vi "DIO.vi"() -> ()   [LabVIEW 2019]
uses:
  <userlib>/DAQNavi Polymorphic VI/create/DAQNavi Create Channel(DO-Digital Output).vi
  <userlib>/DAQNavi Polymorphic VI/create/DAQNavi Create Channel(DI-Digital Input).vi
  <userlib>/DAQNavi Polymorphic VI/create/DAQNavi Create Channel(AI-Voltage).vi
  <vilib>/measure/mamon.llb/Trigger Detection for 1 Channel.vi
  <userlib>/DAQNavi Polymorphic VI/read/DAQNavi Read (Analog 1D DBL NChan 1Samp).vi
  <userlib>/DAQNavi Polymorphic VI/read/DAQNavi Read (Digital 1D U8 NChan 1Samp).vi
  <userlib>/DAQNavi Polymorphic VI/write/DAQNavi Write (Digtial 1D U8 NChan 1Samp).vi
  <vilib>/measure/NI_MAPro.lvlib
panel:
  out "Waveform Chart 2":waveform(i16)(graph)
  out "Waveform Chart":waveform(i16)(graph)
  in  "x":dbl
  out "Elapsed Time (s) 2":dbl caption="Elapsed Time (s)"
  out "output value":dbl
  out "data":dbl[](array[numeric]) format="%.2f"
  out "error out 3":errorcluster
  out "error out 2":errorcluster
  in  "stop":bool
  out "error out":errorcluster
  in  "Dec Disc 30":bool
  in  "Inc Disc 30":bool
  in  "Dec Disc 29":bool
  in  "Inc Disc 29":bool
  in  "Dec Disc 28":bool
  in  "Inc Disc 28":bool
  in  "Dec Disc 27":bool
  in  "Inc Disc 27":bool
  in  "Dec Disc 26":bool
  in  "Inc Disc 26":bool
  out "Auto/Manual Disc 30":bool
  out "Auto/Manual Disc 29":bool
  out "Auto/Manual Disc 28":bool
  out "Auto/Manual Disc 27":bool
  out "Auto/Manual Disc 26":bool
  out "Run/Stop Disc 30":bool
  out "Run/Stop Disc 29":bool
  out "Run/Stop Disc 28":bool
  out "Run/Stop Disc 27":bool
  out "Run/Stop Disc 26":bool
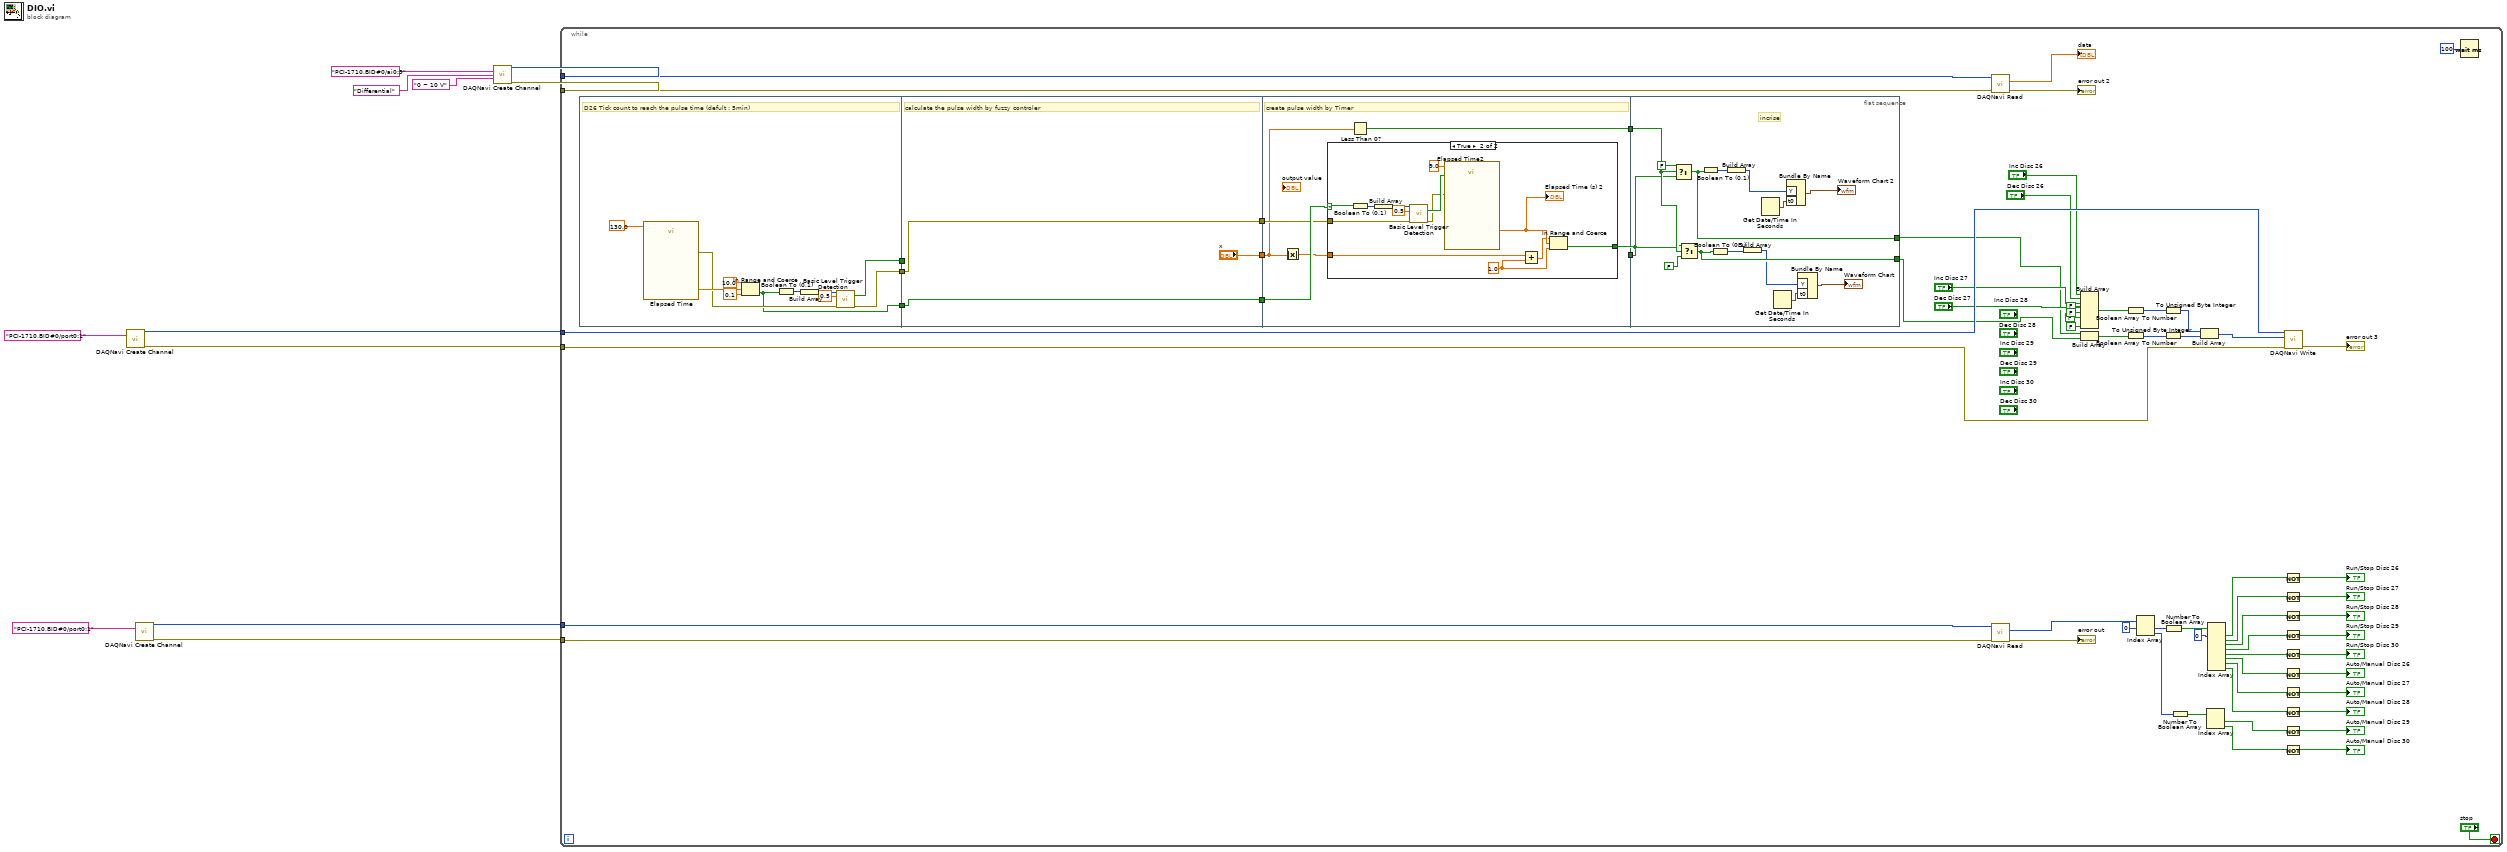
[diagram p0: block diagram]
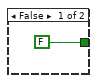
[diagram p2: hidden frame]
diagram:
  n1 = call-poly <userlib>:"DAQNavi Create Channel.vi"("physical channels"="PCI-1710,BID#0/port0:1") -> ("task out"=w11:i32, "error out"=w10:errorcluster)  [unwired: 13 in]
  n2 = call-poly <userlib>:"DAQNavi Create Channel.vi"("physical channels"="PCI-1710,BID#0/port0:1") -> ("task out"=w7:i32, "error out"=w6:errorcluster)  [unwired: 13 in]
  n3 = call-poly <userlib>:"DAQNavi Create Channel.vi"("physical channels"="PCI-1710,BID#0/ai0:9", "signal type"="Differential", "value range"="0 ~ 10 V") -> ("task out"=w2:i32, "error out"=w1:errorcluster)  [unwired: 11 in]
  n4 = while {
    tunnel: w11 -> [w59]
    tunnel: w10 -> [w58]
    tunnel: w7 -> [w57]
    tunnel: w6 -> [w56]
    tunnel: w2 -> [w55]
    tunnel: w1 -> [w54]
    stop <- "stop" stop-if-true
    n5 = flat-sequence {
      tunnel: [w79] -> w29
      tunnel: [w77] -> w28
      tunnel: [w76] -> w27
      tunnel: w29 -> [_]
      tunnel: w28 -> [w88]
      tunnel: [w89] -> w26
      tunnel: w27 -> [w89]
      tunnel: [w88] -> w23
      tunnel: ["x"] -> w22
      tunnel: w26 -> [w95]
      tunnel: [w93] -> w25
      tunnel: [w92] -> w24
      tunnel: w23 -> [w91]
      tunnel: w22 -> [w90]
      tunnel: w25 -> [w121]
      tunnel: w24 -> [w122]
      tunnel: [w118] -> w15
      tunnel: [w114] -> w14
      frame #0 {
        # "D26 Tick count to reach the pulse time (defult : 5min)"
        n6 = call "Elapsed Time"("Time Target (s)"=130.0) -> ("Elapsed Time (s)"=w82:dbl, "error out"=w78:errorcluster)  [unwired: 11 in, 6 out]
        n7 = In Range and Coerce(upper limit=10.0, x=w82, lower limit=0.1) -> (In Range?=w76:bool)  [unwired: 1 out]
        n8 = Boolean To (0,1)(Boolean=w76) -> (0, 1=w86:i16)
        n9 = Build Array(w86) -> (w85:i16[])
        n10 = call-poly <vilib>:"Basic Level Trigger Detection.vi"("signal in"=w85, "level"=0.5, "error in (no error)"=w78) -> ("trigger detected?"=w79:bool, "error out"=w77:errorcluster)  [unwired: 10 in, 1 out]
      }
      frame #1 {
        # "calculate the pulse width by fuzzy controler"
      }
      frame #2 {
        # "create pulse width by Timer"
        n11 = Absolute Value(x=w90) -> (abs(x)=w94:dbl)
        n12 = case shown="True" w95 {
          selector: w95 -> [_ w108]
          tunnel: [FALSE w102] -> w93
          tunnel: w94 -> [_ w101]
          tunnel: w91 -> [_ w98]
          frame False {
          }
          frame True {
            w100 = 1.0 ("lower limit")
            n13 = Boolean To (0,1)(Boolean=w108) -> (0, 1=w107:i16)
            n14 = Build Array(w107) -> (w106:i16[])
            n15 = call-poly <vilib>:"Basic Level Trigger Detection.vi"("signal in"=w106, "level"=0.5, "error in (no error)"=w98) -> ("trigger detected?"=w104:bool, "error out"=w97:errorcluster)  [unwired: 10 in, 1 out]
            n16 = call "Elapsed Time2"("Time Target (s)"=9.0, "Reset"=w104, "error in (no error)"=w97) -> ("Elapsed Time (s)"=w103:dbl)  [unwired: 9 in, 7 out]
            "Elapsed Time (s) 2" <- w103
            n17 = Add(x=w101, y=w100) -> (x+y=w99:dbl)
            n18 = In Range and Coerce(upper limit=w99, x=w103, lower limit=w100) -> (In Range?=w102:bool)  [unwired: 1 out]
          }
        }
        n19 = Less Than 0?(x=w90) -> (x < 0?=w92:bool)
      }
      frame #3 {
        # "incrise"
        n20 = Select(t=FALSE, s=w122, f=w121) -> (s? t:f=w118:bool)
        n21 = Select(t=w121, s=w122, f=FALSE ("t")) -> (s? t:f=w114:bool)
        n22 = Boolean To (0,1)(Boolean=w118) -> (0, 1=w117:i16)
        n23 = Boolean To (0,1)(Boolean=w114) -> (0, 1=w115:i16)
        n24 = Build Array(w117) -> (w116:i16[])
        n25 = Build Array(w115) -> (w112:i16[])
        n26 = Get Date/Time In Seconds() -> (seconds since 1Jan1904=w119:timestamp)
        n27 = Get Date/Time In Seconds() -> (seconds since 1Jan1904=w113:timestamp)
        n28 = Bundle By Name("Y"=w116, "t0"=w119) -> (→"Waveform Chart 2":waveform(i16))  [unwired: 1 in]
        n29 = Bundle By Name("Y"=w112, "t0"=w113) -> (→"Waveform Chart":waveform(i16))  [unwired: 1 in]
      }
    }
    n30 = call-poly <userlib>:"DAQNavi Read.vi"("error in (no error)"=w54, "task in"=w55) -> ("error out"=→"error out 2":errorcluster, "data"=→"data":dbl[])  [unwired: 7 in, 1 out]
    n31 = call-poly <userlib>:"DAQNavi Read.vi"("error in (no error)"=w56, "task in"=w57) -> ("error out"=→"error out":errorcluster, "data"=w75:u8[])  [unwired: 7 in, 1 out]
    n32 = Build Array("Inc Disc 26", "Dec Disc 26", "Inc Disc 27", "Dec Disc 27", FALSE ("element"), FALSE ("element"), FALSE ("element"), FALSE ("element")) -> (w69:bool[])
    n33 = Build Array(w15, w14) -> (w68:bool[])
    n34 = Boolean Array To Number(Boolean array=w69) -> (number=w67:u32)
    n35 = Boolean Array To Number(Boolean array=w68) -> (number=w65:u32)
    n36 = Index Array(array=w75, index #1=0 ("index")) -> (element #1=w62:u8, element #2=w73:u8)  [unwired: 1 in]
    n37 = To Unsigned Byte Integer(number=w67) -> (unsigned 8bit integer=w66:u8)
    n38 = To Unsigned Byte Integer(number=w65) -> (unsigned 8bit integer=w64:u8)
    n39 = Number To Boolean Array(number=w62) -> (Boolean array=w72:bool[])
    n40 = Number To Boolean Array(number=w73) -> (Boolean array=w70:bool[])
    n41 = Build Array(w66, w64) -> (w63:u8[])
    n42 = Index Array(array=w70) -> (element #1=w36:bool, element #2=w35:bool)  [unwired: 2 in]
    n43 = Index Array(array=w72, index #1=0 ("index")) -> (element #1=w47:bool, element #2=w45:bool, element #3=w44:bool, element #4=w43:bool, element #5=w49:bool, element #6=w39:bool, element #7=w38:bool, element #8=w37:bool)  [unwired: 7 in]
    n44 = Not(x=w47) -> (.not. x?=→"Run/Stop Disc 26":bool)
    n45 = Not(x=w45) -> (.not. x?=→"Run/Stop Disc 27":bool)
    n46 = Not(x=w44) -> (.not. x?=→"Run/Stop Disc 28":bool)
    n47 = Not(x=w43) -> (.not. x?=→"Run/Stop Disc 29":bool)
    n48 = Not(x=w49) -> (.not. x?=→"Run/Stop Disc 30":bool)
    n49 = Not(x=w39) -> (.not. x?=→"Auto/Manual Disc 26":bool)
    n50 = Not(x=w38) -> (.not. x?=→"Auto/Manual Disc 27":bool)
    n51 = Not(x=w37) -> (.not. x?=→"Auto/Manual Disc 28":bool)
    n52 = Not(x=w36) -> (.not. x?=→"Auto/Manual Disc 29":bool)
    n53 = Not(x=w35) -> (.not. x?=→"Auto/Manual Disc 30":bool)
    n54 = call-poly <userlib>:"DAQNavi Write.vi"("error in (no error)"=w58, "data"=w63, "task in"=w59) -> ("error out"=→"error out 3":errorcluster)  [unwired: 6 in, 2 out]
    n55 = Wait (ms)(milliseconds to wait=u32 100) -> ()  [unwired: 1 out]
  }
